vi "Parallel - Interleaved.vi"(7 "Name":string="Parallel", 9 "Always Repeat First Node":bool, 10 "Status Calculation":T1, 11 "Nodes":refnum<class "abs_Node.lvclass">[](array[class])) -> (3 "Node":refnum<class "abs_Node.lvclass">)   [LabVIEW 2021, in "BT.lvlib"]
uses:
  BT.lvlib
  abs_Node/abs_Node.lvclass
  abs_Parallel/Support/Status Calculation.ctl
  Parallel_Interleaved/Parallel_Interleaved.lvclass
  C:/Users/Tim/Documents/LabVIEW/2021/Behaviour Tree/abs_Composite/abs_Composite.lvclass
  C:/Users/Tim/Documents/LabVIEW/2021/Behaviour Tree/abs_Node/abs_Node.lvclass
  C:/Users/Tim/Documents/LabVIEW/2021/Behaviour Tree/abs_Parallel/abs_Parallel.lvclass
  abs_Composite/abs_Composite.lvclass/abs_Composite.ctl
  abs_Node/abs_Node.lvclass/abs_Node.ctl
  abs_Parallel/abs_Parallel.lvclass/abs_Parallel.ctl
  Parallel_Interleaved/Parallel_Interleaved.lvclass/Parallel_Interleaved.ctl
  abs_Composite/Properties/Write Nodes.vi
  abs_Node/Properties/Write Name.vi
  abs_Parallel/Properties/Write Status Calculation.vi
  Parallel_Interleaved/Properties/Write Always Repeat First Node.vi
  abs_Parallel/abs_Parallel.lvclass
panel:
  # "The first node can be used for tick timing cpu overhead."
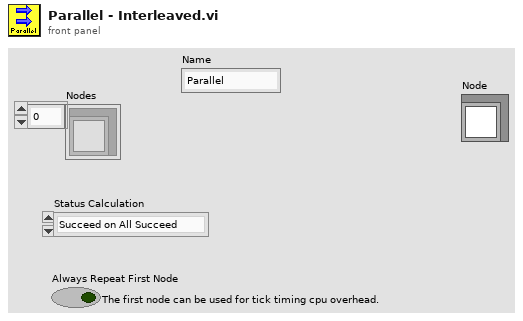
[diagram p1: front panel]
types:
  T1 = typedef "BT.lvlib/abs_Parallel.lvclass/Status Calculation.ctl" = enum16{"Succeed on All Succeed", "Failure on All Failure", "Succeed on Any Succeed", "Failure on Any Failure"}
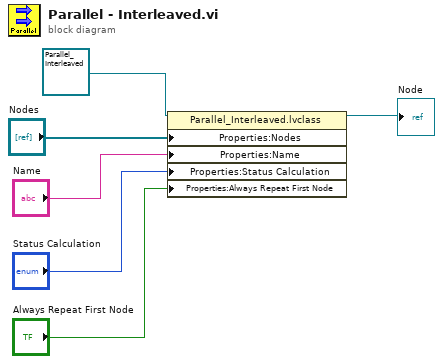
[diagram p0: block diagram]
diagram:
  n1 = property class="Parallel_Interleaved.lvclass"(reference=refnum<class "Parallel_Interleaved.lvclass"> refnum ("BT.lvlib:Parallel_Interleaved.lvclass"), "Properties:Nodes"="Nodes", "Properties:Name"="Name", "Properties:Status Calculation"="Status Calculation", "Properties:Always Repeat First Node"="Always Repeat First Node") -> (reference out=→"Node":refnum<class "Parallel_Interleaved.lvclass">)  [unwired: 1 in, 1 out]
